vi "Example 1.vi"() -> ()   [LabVIEW 2016]
uses:
  listbox/listbox.lvclass
  LNK/Copy/Copy.lvclass
  E:/OMRON Motion measurement/ListboxMenu/LNK/Parent Class/Menu.lvclass
  LNK/Delete/Delete.lvclass
  LNK/UP/UP.lvclass
  LNK/Down/Down.lvclass
  LNK/Parent Class/Menu.lvclass
  listbox/listbox.lvclass/listbox.ctl
panel:
  in  "停止":bool
  in  "多列列表框":i32(listbox)=4
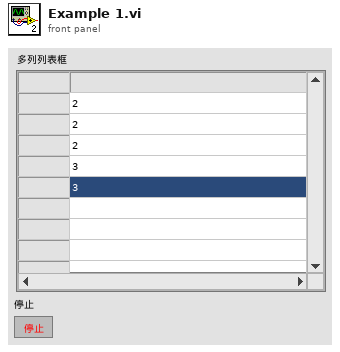
[diagram p1: front panel]
types:
  T1 = typedef "LVPoint32TypeDef.ctl" = cluster{"Horizontal":i32, "Vertical":i32}
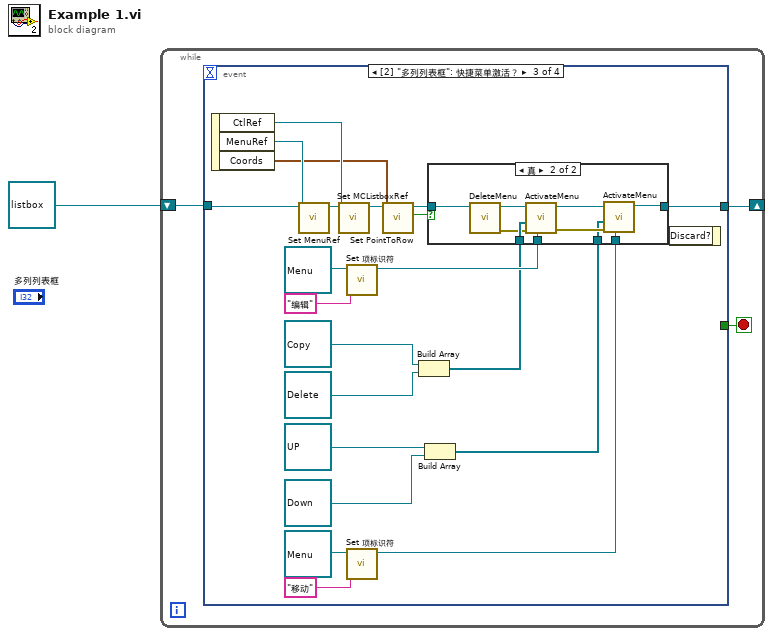
[diagram p0: block diagram]
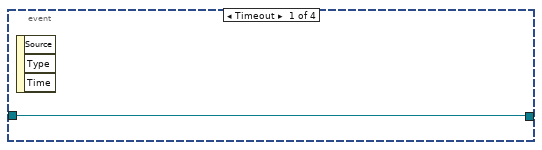
[diagram p2: hidden frame]
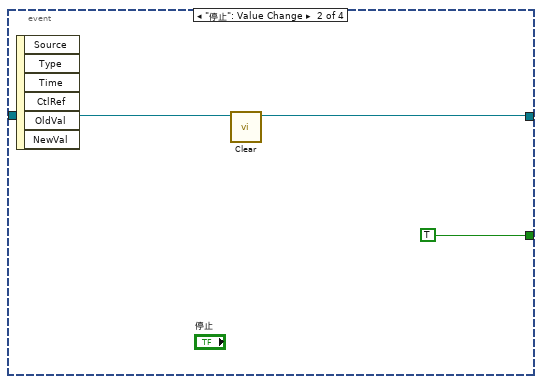
[diagram p3: hidden frame]
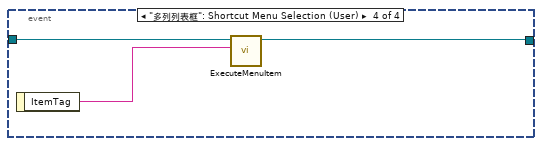
[diagram p5: hidden frame]
diagram:
  n1 = while {
    shift-right: [w2] -> _
    shift-left: refnum<class "listbox.lvclass"> refnum ("listbox.lvclass") -> [w3]
    stop <- w4 stop-if-true
    n2 = event shown="[2] \"多列列表框\": 快捷菜单激活？" {
      selector: _ -> [_ _ _ _]
      dyn-events: _ -> [_ _ _ _]
      timeout: _ -> [_ _ _ _]
      tunnel: [_ TRUE _ _] -> w4
      tunnel: w3 -> [w5 w7 w29 w43]
      tunnel: [w5 w6 w25 w42] -> w2
      event Timeout {
        n3 = event-data() -> ()  [unwired: 1 in, 3 out]
      }
      event "停止": Value Change {
        n4 = event-data() -> ()  [unwired: 1 in, 6 out]
        n5 = call "Clear.vi"("listbox 输入"=w7) -> ("listbox 输出"=w6:refnum<class "listbox.lvclass">)  [unwired: 9 in, 1 out]
      }
      event "多列列表框": Shortcut Menu Activation? {
        n6 = event-data() -> ("CtlRef"=w24:refnum<vi>, "MenuRef"=w28:refnum<k9>, "Coords"=w22:T1)  [unwired: 1 in]
        n7 = call "Set MenuRef.vi"("MenuRef"=w28, "listbox in"=w29) -> ("listbox out"=w27:refnum<class "listbox.lvclass">)  [unwired: 9 in]
        n8 = call "Set MCListboxRef.vi"("MCListboxRef"=w24, "listbox in"=w27) -> ("listbox out"=w26:refnum<class "listbox.lvclass">)  [unwired: 9 in]
        n9 = call "Set 项标识符.vi"("项标识符"="编辑", "LNK in"=refnum<class "Menu.lvclass"> refnum ("Menu.lvclass")) -> ("LNK out"=w12:refnum<class "Menu.lvclass">)  [unwired: 9 in]
        n10 = call "Set 项标识符.vi"("项标识符"="移动", "LNK in"=refnum<class "Menu.lvclass"> refnum ("Menu.lvclass")) -> ("LNK out"=w9:refnum<class "Menu.lvclass">)  [unwired: 9 in]
        n11 = call "Set PointToRow.vi"("坐标"=w22, "listbox 输入"=w26) -> ("边界内？"=w21:bool, "listbox 输出"=w23:refnum<class "listbox.lvclass">)  [unwired: 7 in, 1 out]
        n12 = Build Array(refnum<class "Copy.lvclass"> refnum ("Copy.lvclass"), refnum<class "Delete.lvclass"> refnum ("Delete.lvclass")) -> (w11:refnum<class "Menu.lvclass">[])
        n13 = Build Array(refnum<class "UP.lvclass"> refnum ("UP.lvclass"), refnum<class "Down.lvclass"> refnum ("Down.lvclass")) -> (w10:refnum<class "Menu.lvclass">[])
        n14 = case shown="真" w21 {
          tunnel: w11 -> [_ w40]
          tunnel: [w30 w35] -> w25
          tunnel: w23 -> [w30 w37]
          tunnel: w12 -> [_ w36]
          tunnel: w9 -> [_ w32]
          tunnel: w10 -> [_ w31]
          frame False {
          }
          frame True {
            n15 = call "DeleteMenu.vi"("listbox 输入"=w37) -> ("error out"=w38:errorcluster, "listbox 输出"=w39:refnum<class "listbox.lvclass">)  [unwired: 9 in]
            n16 = call "ActivateMenu.vi"("Menu.lvclass"=w36, "error in (no error)"=w38, "MenuClassArray"=w40, "listbox 输入"=w39) -> ("error out"=w33:errorcluster, "listbox 输出"=w34:refnum<class "listbox.lvclass">)  [unwired: 6 in]
            n17 = call "ActivateMenu.vi"("Menu.lvclass"=w32, "error in (no error)"=w33, "MenuClassArray"=w31, "listbox 输入"=w34) -> ("listbox 输出"=w35:refnum<class "listbox.lvclass">)  [unwired: 6 in, 1 out]
          }
        }
        n18 = event-data() -> ()  [unwired: 2 in, 1 out]
      }
      event "多列列表框": Shortcut Menu Selection (User) {
        n19 = event-data() -> ("ItemTag"=w41:string)  [unwired: 1 in]
        n20 = call "ExecuteMenuItem.vi"("项标识符"=w41, "listbox 输入"=w43) -> ("listbox 输出"=w42:refnum<class "listbox.lvclass">)  [unwired: 8 in, 1 out]
      }
    }
  }
